vi "Calculate f for settling time calc.vi"(4 "Sampling Freq (Hz)":dbl format="%#_13g", 5 "Scope Waveform":dbl[](array[numeric])) -> (1 "Frequency 'f'":dbl)   [LabVIEW 2020, in "LDO Line Transient.lvlib"]
uses:
  LDO Line Transient.lvlib
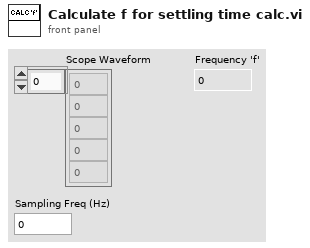
[diagram p1: front panel]
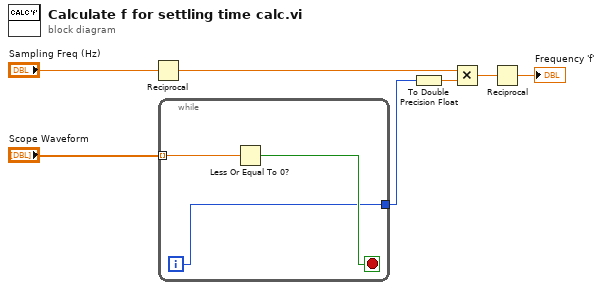
[diagram p0: block diagram]
diagram:
  n1 = Reciprocal(x="Sampling Freq (Hz)") -> (1/x=w5:dbl)
  n2 = while {
    tunnel: "Scope Waveform" -> [w10] mode=indexing
    tunnel: [w8] -> w4
    i -> [w8]
    stop <- w9 stop-if-true
    n3 = Less Or Equal To 0?(x=w10) -> (x <= 0?=w9:bool)
  }
  n4 = To Double Precision Float(number=w4) -> (double precision float=w3:dbl)
  n5 = Multiply(x=w5, y=w3) -> (x*y=w2:dbl)
  n6 = Reciprocal(x=w2) -> (1/x=→"Frequency 'f'":dbl)
